vi "Celestial GOTO GUI.vi"() -> ()   [LabVIEW 2017]
uses:
  CaseEnum.ctl
  EventCase.ctl
  <vilib>/Instr/_visa.llb/VISA Configure Serial Port (Instr).vi
panel:
  out "DEC Angular Degrees":dbl[](array[numeric]) format="%#_4g"
  out "RA Angular Degrees":dbl[](array[numeric]) format="%#_4g"
  out "Source Coordinates RA/DE":T1
  in  "Source Target":u32(ring) items=["Mirach", "Mirphak", "Deneb", "Vega", "Sadr", "NGC6960", "M31", "M27", "M33", "M45", ""]
  in  "DEC-":bool
  in  "DEC+":bool
  in  "RA-":bool
  in  "RA+":bool
  in  "GOTO Destination":bool
  in  "VISA resource name":refnum<visa-resource-name>
  out "Serial Response":string
  out "Error Out":errorcluster
  out "Coordinate Difference (degrees)":cluster{"RA Degrees":dbl, "DE Degrees":dbl} {"DE Degrees" format="%#_3g"; "RA Degrees" format="%#_3g"}
  out "Destination Coordinates RA/DE":T1
  in  "Destination Target":u32(ring) items=["Mirach", "Mirphak", "Deneb", "Vega", "Sadr", "NGC6960", "M31", "M27", "M33", "M45", ""]
  in  "Stop Button":bool
  in  "Cluster":T2 {"Degrees to Move" format="%#_2g"}
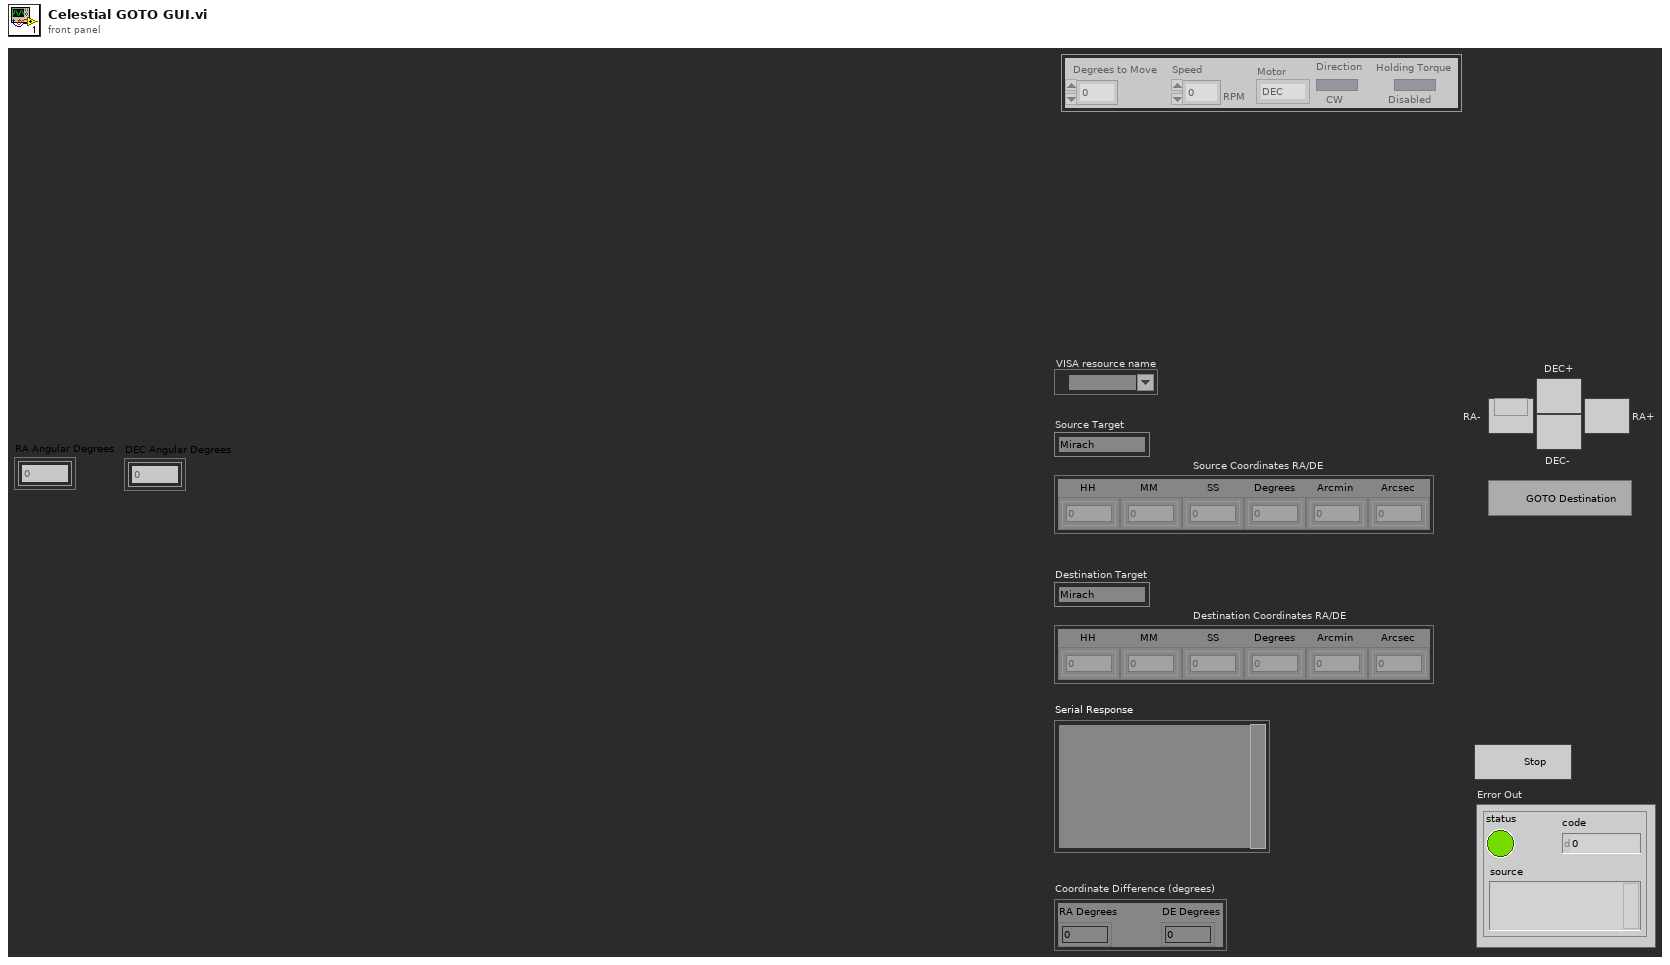
[diagram p1: front panel]
types:
  T1 = cluster{"HH":i32[], "MM":i32[], "SS":i32[], "Degrees":i32[], "Arcmin":i32[], "Arcsec":i32[]}
  T2 = cluster{"Degrees to Move":dbl, "Speed":i32, "Motor":enum16{"DEC", "RA"}, "Direction":bool, "Holding Torque":bool}
  T3 = typedef "CaseEnum.ctl" = enum16{"Default", "Parse Database", "Compute Coordinate Difference", "Move RA Motor", "Wait", "Move DEC Motor", "RA-", "RA+", "DEC-", "DEC+"}
  T4 = typedef "EventCase.ctl" = enum16{"Event", "Serial Write", "Wait", "Serial Read", "Stop"}
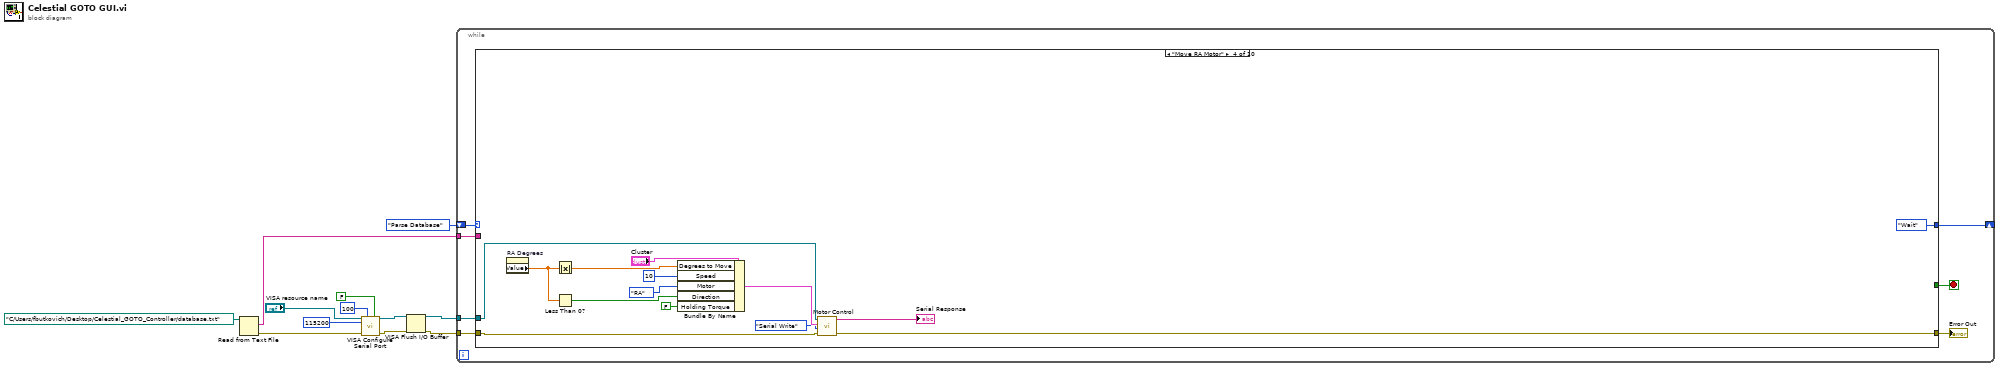
[diagram p0: block diagram]
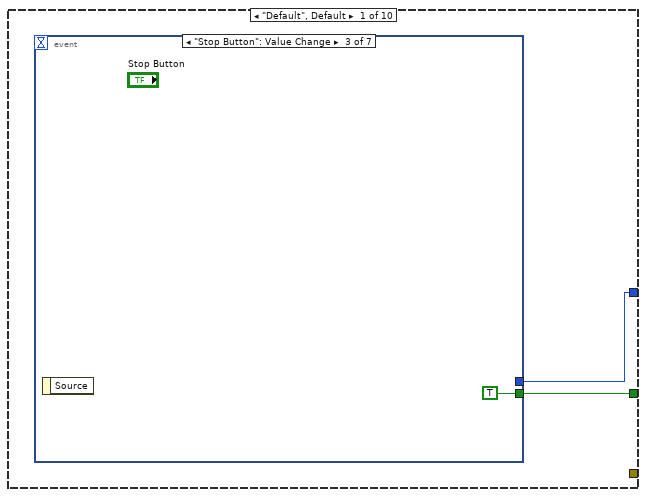
[diagram p2: hidden frame]
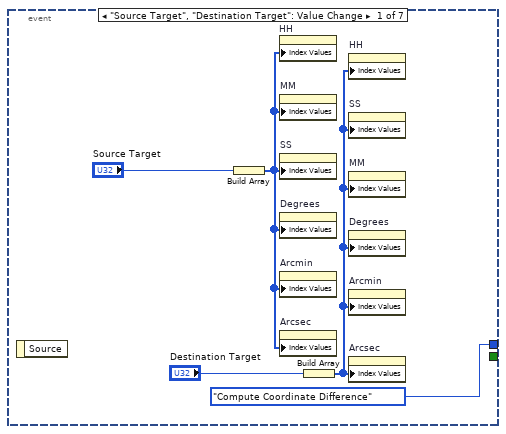
[diagram p3: hidden frame]
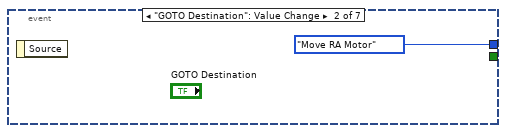
[diagram p4: hidden frame]
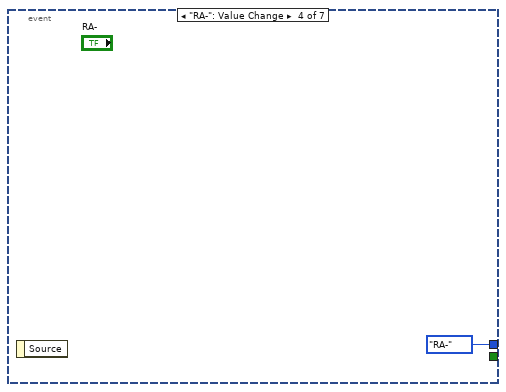
[diagram p5: hidden frame]
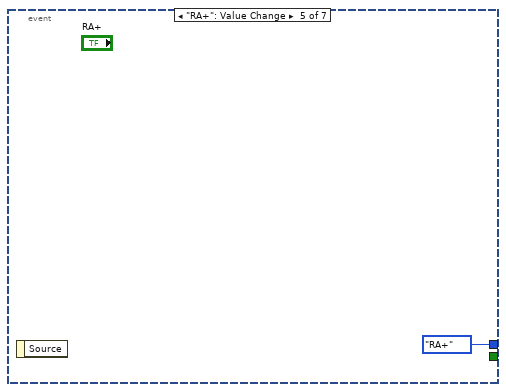
[diagram p6: hidden frame]
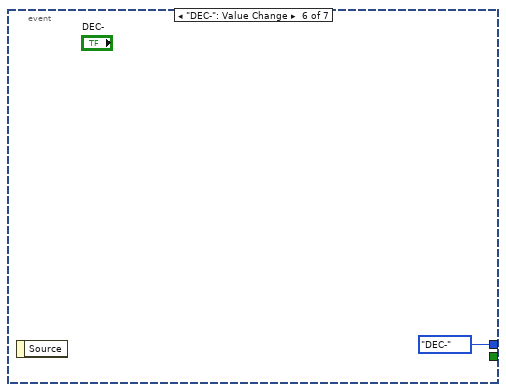
[diagram p7: hidden frame]
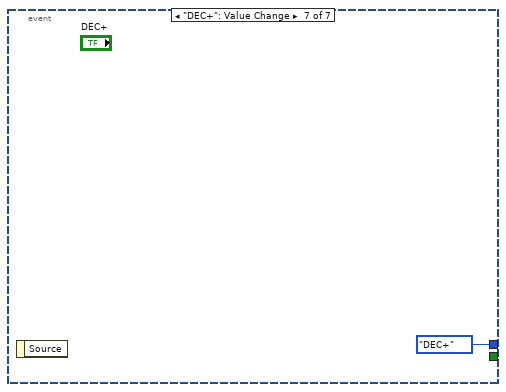
[diagram p8: hidden frame]
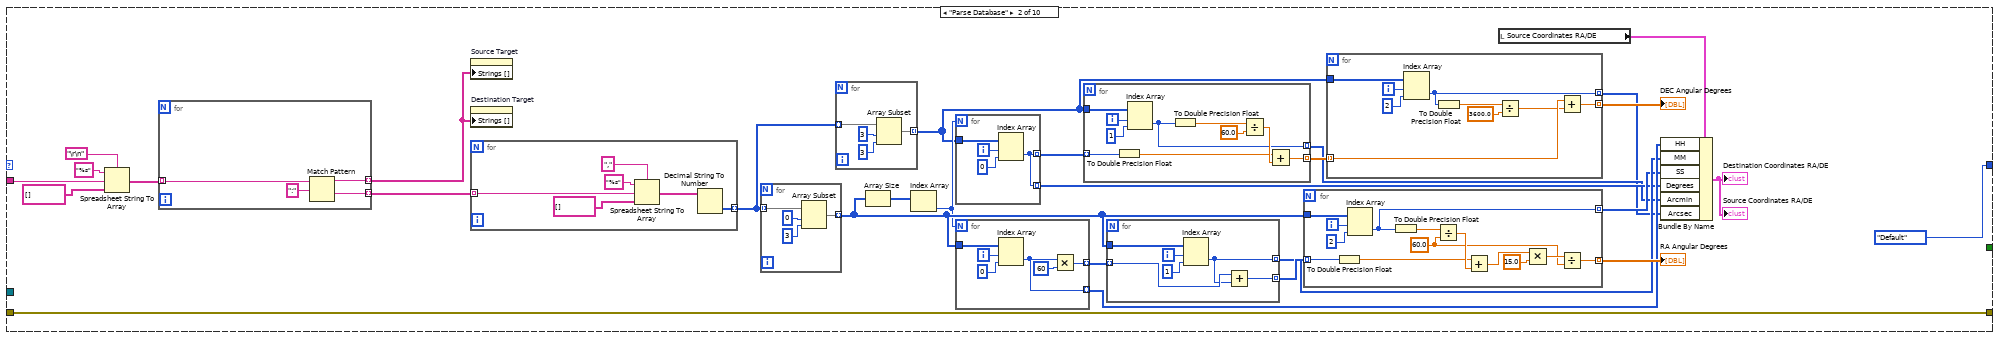
[diagram p9: hidden frame]
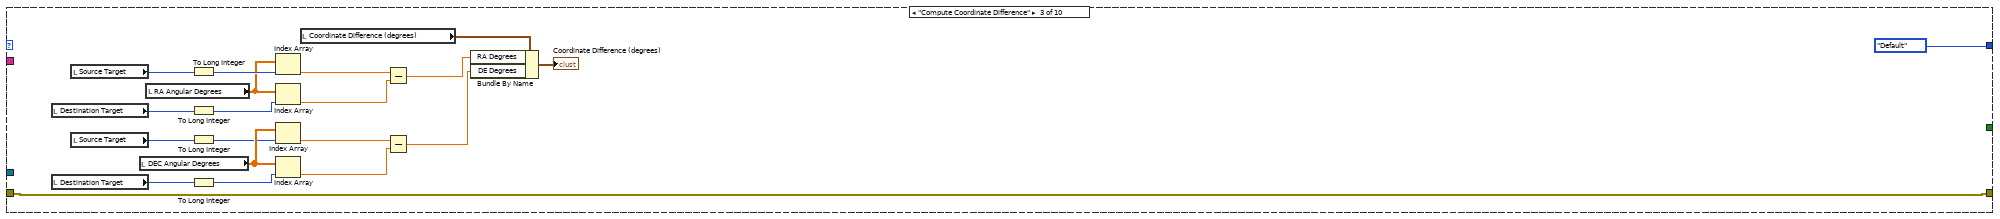
[diagram p10: hidden frame]
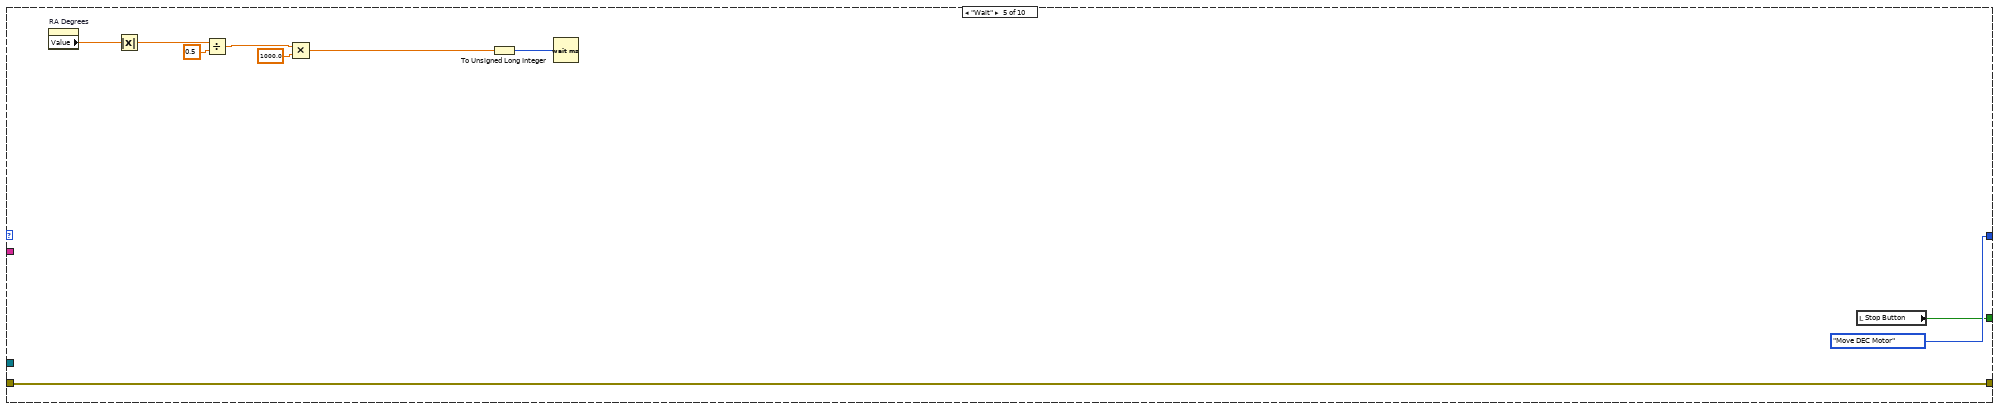
[diagram p11: hidden frame]
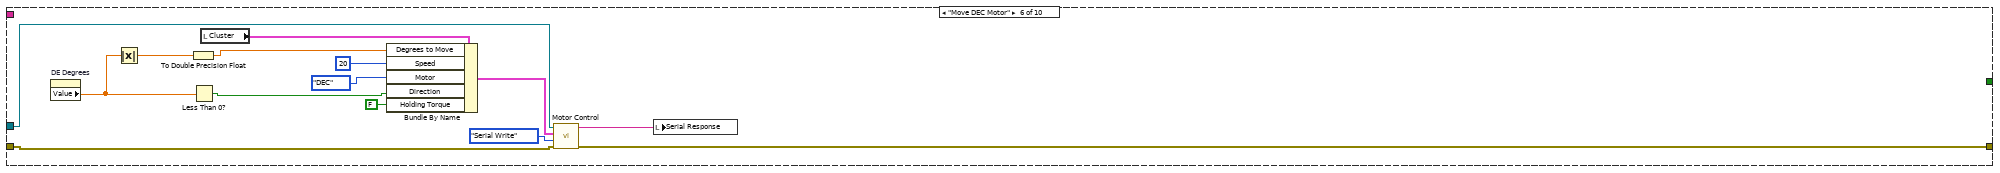
[diagram p12: hidden frame]
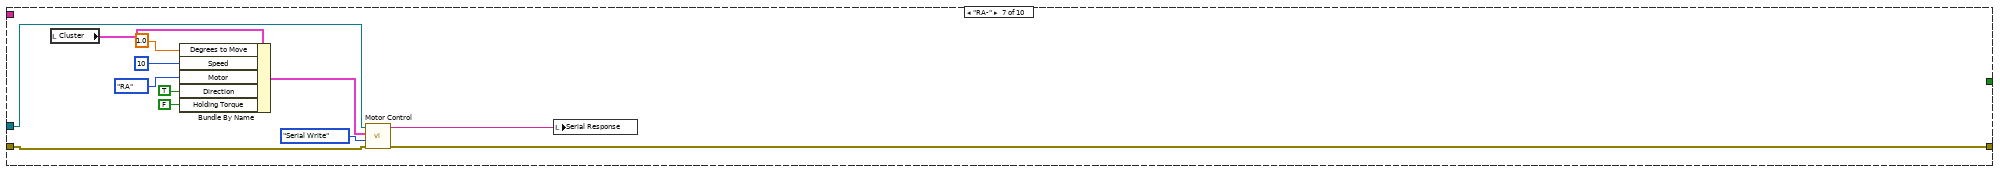
[diagram p13: hidden frame]
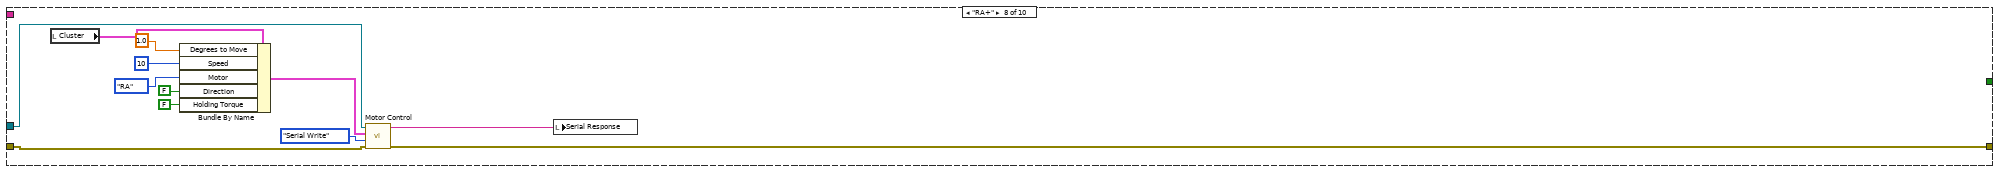
[diagram p14: hidden frame]
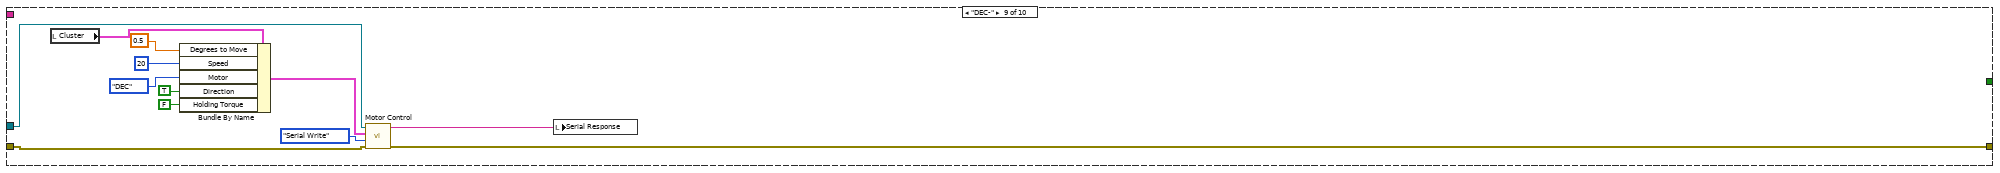
[diagram p15: hidden frame]
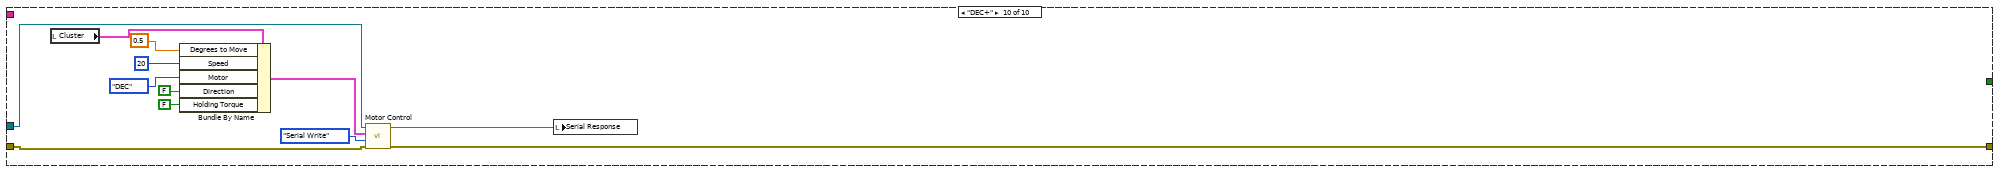
[diagram p16: hidden frame]
diagram:
  n1 = Read from Text File(file (use dialog)=path "C:/Users/fbutkovich/Desktop/Celestial_GOTO_Controller/database.txt" ("file path (use dialog)")) -> (text=w10:string, error out=w5:errorcluster)  [unwired: 3 in, 2 out]
  n2 = call-poly "VISA Configure Serial Port"("VISA resource name"="VISA resource name", "timeout (10sec)"=u32 100, "Enable Termination\nChar (T)"=FALSE, "baud rate (9600)"=u32 115200, "error in (no error)"=w5) -> ("VISA resource name out"=w6:refnum<visa-resource-name>, "error out"=w2:errorcluster)  [unwired: 9 in]
  n3 = VISA Flush I/O Buffer(VISA resource name=w6, error in (no error)=w2) -> (VISA resource name out=w3:refnum<visa-resource-name>, error out=w1:errorcluster)  [unwired: 1 in]
  n4 = while {
    tunnel: w10 -> [w17]
    tunnel: w1 -> [w15]
    shift-right: [w18] -> _
    shift-left: CaseEnum."Parse Database" -> [w19]
    tunnel: w3 -> [w13]
    stop <- w16 stop-if-true
    n5 = case shown="\"Move RA Motor\"" w19 {
      tunnel: [w21 CaseEnum."Default" CaseEnum."Default" CaseEnum."Wait" CaseEnum."Move DEC Motor" _ _ _ _ _] -> w18
      tunnel: w17 -> [_ w54 _ _ _ _ _ _ _ _]
      tunnel: [w20 _ _ _ w162 _ _ _ _ _] -> w16
      tunnel: [_ w59 w127 w159 w161 w184 w190 w197 w210 w224] -> w14
      tunnel: w15 -> [_ w59 w127 w148 w161 w173 w191 w201 w211 w225]
      tunnel: w13 -> [_ _ _ w150 _ w175 w192 w202 w212 w226]
      frame "Default", Default {
        n6 = event shown="[2] \"Stop Button\": Value Change" {
          selector: _ -> [_ _ _ _ _ _ _]
          dyn-events: _ -> [_ _ _ _ _ _ _]
          timeout: _ -> [_ _ _ _ _ _ _]
          tunnel: [CaseEnum."Compute Coordinate Difference" CaseEnum."Move RA Motor" _ CaseEnum."RA-" CaseEnum."RA+" CaseEnum."DEC-" CaseEnum."DEC+"] -> w21
          tunnel: [_ _ TRUE _ _ _ _] -> w20
          event "Source Target", "Destination Target": Value Change {
            n7 = event-data() -> ()  [unwired: 1 in, 1 out]
            n8 = Build Array("Source Target") -> (w22:u32[])
            n9 = property on="HH" class="Arr (strict)"("Index Values"=w22) -> ()  [unwired: 2 in, 2 out]
            n10 = property on="MM" class="Arr (strict)"("Index Values"=w22) -> ()  [unwired: 2 in, 2 out]
            n11 = property on="SS" class="Arr (strict)"("Index Values"=w22) -> ()  [unwired: 2 in, 2 out]
            n12 = property on="Degrees" class="Arr (strict)"("Index Values"=w22) -> ()  [unwired: 2 in, 2 out]
            n13 = property on="Arcmin" class="Arr (strict)"("Index Values"=w22) -> ()  [unwired: 2 in, 2 out]
            n14 = property on="Arcsec" class="Arr (strict)"("Index Values"=w22) -> ()  [unwired: 2 in, 2 out]
            n15 = Build Array("Destination Target") -> (w23:u32[])
            n16 = property on="HH" class="Arr (strict)"("Index Values"=w23) -> ()  [unwired: 2 in, 2 out]
            n17 = property on="SS" class="Arr (strict)"("Index Values"=w23) -> ()  [unwired: 2 in, 2 out]
            n18 = property on="MM" class="Arr (strict)"("Index Values"=w23) -> ()  [unwired: 2 in, 2 out]
            n19 = property on="Degrees" class="Arr (strict)"("Index Values"=w23) -> ()  [unwired: 2 in, 2 out]
            n20 = property on="Arcmin" class="Arr (strict)"("Index Values"=w23) -> ()  [unwired: 2 in, 2 out]
            n21 = property on="Arcsec" class="Arr (strict)"("Index Values"=w23) -> ()  [unwired: 2 in, 2 out]
          }
          event "GOTO Destination": Value Change {
            n22 = event-data() -> ()  [unwired: 1 in, 1 out]
          }
          event "Stop Button": Value Change {
            n23 = event-data() -> ()  [unwired: 1 in, 1 out]
          }
          event "RA-": Value Change {
            n24 = event-data() -> ()  [unwired: 1 in, 1 out]
          }
          event "RA+": Value Change {
            n25 = event-data() -> ()  [unwired: 1 in, 1 out]
          }
          event "DEC-": Value Change {
            n26 = event-data() -> ()  [unwired: 1 in, 1 out]
          }
          event "DEC+": Value Change {
            n27 = event-data() -> ()  [unwired: 1 in, 1 out]
          }
        }
      }
      frame "Parse Database" {
        n28 = Spreadsheet String To Array(delimiter (Tab)="\r\n", format string="%s", spreadsheet string=w54, array type (2D Dbl)=string[] []) -> (array=w55:string[])
        n29 = for {
          tunnel: w55 -> [w126] mode=indexing
          tunnel: [w124] -> w41 mode=indexing
          tunnel: [w123] -> w53 mode=indexing
          n30 = Match Pattern(string=w126, regular expression=":") -> (before substring=w123:string, after substring=w124:string)  [unwired: 1 in, 2 out]
        }
        n31 = property on="Source Target" class="Ring (strict)"("Strings []"=w53) -> ()  [unwired: 2 in, 2 out]
        n32 = property on="Destination Target" class="Ring (strict)"("Strings []"=w53) -> ()  [unwired: 2 in, 2 out]
        n33 = for {
          tunnel: [w118] -> w52 mode=indexing
          tunnel: w41 -> [w117] mode=indexing
          n34 = Spreadsheet String To Array(delimiter (Tab)=",", format string="%s", spreadsheet string=w117, array type (2D Dbl)=string[] []) -> (array=w119:string[])
          n35 = Decimal String To Number(string=w119) -> (number=w118:i32[])  [unwired: 2 in, 1 out]
        }
        n36 = for {
          tunnel: w52 -> [w116] mode=indexing
          tunnel: [w115] -> w49 mode=indexing
          n37 = Array Subset(array=w116, index=0, length=3) -> (w115:i32[])
        }
        n38 = for {
          tunnel: w52 -> [w112] mode=indexing
          tunnel: [w111] -> w44 mode=indexing
          n39 = Array Subset(array=w112, index=3, length=3) -> (w111:i32[])
        }
        n40 = Array Size(array=w49) -> (size(s)=w51:i32[])
        n41 = Index Array(array=w51) -> (element=w45:i32)  [unwired: 1 in]
        n42 = for {
          N: w45 -> [_]
          tunnel: w44 -> [w83]
          tunnel: [w80] -> w46 mode=indexing
          tunnel: [w80] -> w36 mode=indexing
          i -> [w82]
          n43 = Index Array(array=w83, index (row)=w82, index (col)=0 ("disabled index (col)")) -> (element=w80:i32)
        }
        n44 = for {
          N: w45 -> [_]
          tunnel: w49 -> [w108]
          tunnel: [w104] -> w50 mode=indexing
          tunnel: [w103] -> w39 mode=indexing
          i -> [w107]
          n45 = Index Array(array=w108, index (row)=w107, index (col)=0 ("disabled index (col)")) -> (element=w103:i32)
          n46 = Multiply(x=w103, y=60) -> (x*y=w104:i32)
        }
        n47 = for {
          tunnel: w44 -> [w78]
          tunnel: w46 -> [w77] mode=indexing
          tunnel: [w76] -> w43 mode=indexing
          tunnel: [w70] -> w35 mode=indexing
          i -> [w75]
          n48 = To Double Precision Float(number=w77) -> (double precision float=w71:dbl)
          n49 = Index Array(array=w78, index (row)=w75, index (col)=1) -> (element=w70:i32)
          n50 = To Double Precision Float(number=w70) -> (double precision float=w73:dbl)
          n51 = Divide(x=w73, y=60.0) -> (x/y=w72:dbl)
          n52 = Add(x=w71, y=w72) -> (x+y=w76:dbl)
        }
        n53 = for {
          tunnel: w49 -> [w101]
          tunnel: w50 -> [w100] mode=indexing
          tunnel: [w99] -> w48 mode=indexing
          tunnel: [w97] -> w38 mode=indexing
          i -> [w98]
          n54 = Index Array(array=w101, index (row)=w98, index (col)=1) -> (element=w97:i32)
          n55 = Add(x=w100, y=w97) -> (x+y=w99:i32)
        }
        n56 = for {
          tunnel: w49 -> [w95]
          tunnel: w48 -> [w94] mode=indexing
          tunnel: [w85] -> w47 mode=indexing
          tunnel: [w84] -> w37 mode=indexing
          i -> [w93]
          w86 = 60.0 ("y")
          n57 = To Double Precision Float(number=w94) -> (double precision float=w90:dbl)
          n58 = Index Array(array=w95, index (row)=w93, index (col)=2) -> (element=w84:i32)
          n59 = To Double Precision Float(number=w84) -> (double precision float=w92:dbl)
          n60 = Divide(x=w92, y=w86) -> (x/y=w91:dbl)
          n61 = Add(x=w90, y=w91) -> (x+y=w89:dbl)
          n62 = Multiply(x=w89, y=15.0) -> (x*y=w87:dbl)
          n63 = Divide(x=w87, y=w86) -> (x/y=w85:dbl)
        }
        "RA Angular Degrees" <- w47
        n64 = for {
          tunnel: w44 -> [w68]
          tunnel: w43 -> [w67] mode=indexing
          tunnel: [w66] -> w42 mode=indexing
          tunnel: [w61] -> w33 mode=indexing
          i -> [w65]
          n65 = Index Array(array=w68, index (row)=w65, index (col)=2) -> (element=w61:i32)
          n66 = To Double Precision Float(number=w61) -> (double precision float=w63:dbl)
          n67 = Divide(x=w63, y=3600.0) -> (x/y=w62:dbl)
          n68 = Add(x=w67, y=w62) -> (x+y=w66:dbl)
        }
        "DEC Angular Degrees" <- w42
        n69 = local read "Source Coordinates RA/DE"() -> (w40:T1)
        n70 = Bundle By Name(cluster=w40, "HH"=w39, "MM"=w38, "SS"=w37, "Degrees"=w36, "Arcmin"=w35, "Arcsec"=w33) -> (→"Destination Coordinates RA/DE" →"Source Coordinates RA/DE":T1)
      }
      frame "Compute Coordinate Difference" {
        n71 = local read "Destination Target"() -> (w138:u32)
        n72 = local read "Destination Target"() -> (w141:u32)
        n73 = local read "Source Target"() -> (w143:u32)
        n74 = local read "Source Target"() -> (w132:u32)
        n75 = local read "DEC Angular Degrees"() -> (w133:dbl[])
        n76 = local read "RA Angular Degrees"() -> (w136:dbl[])
        n77 = To Long Integer(number=w143) -> (32bit integer=w139:i32)
        n78 = To Long Integer(number=w138) -> (32bit integer=w137:i32)
        n79 = To Long Integer(number=w132) -> (32bit integer=w131:i32)
        n80 = To Long Integer(number=w141) -> (32bit integer=w140:i32)
        n81 = Index Array(array=w136, index=w139) -> (element=w142:dbl)
        n82 = Index Array(array=w136, index=w137) -> (element=w135:dbl)
        n83 = Index Array(array=w133, index=w131) -> (element=w130:dbl)
        n84 = Index Array(array=w133, index=w140) -> (element=w129:dbl)
        n85 = local read "Coordinate Difference (degrees)"() -> (w145:cluster{"RA Degrees":dbl, "DE Degrees":dbl})
        n86 = Subtract(x=w142, y=w135) -> (x-y=w134:dbl)
        n87 = Subtract(x=w130, y=w129) -> (x-y=w128:dbl)
        n88 = Bundle By Name(cluster=w145, "RA Degrees"=w134, "DE Degrees"=w128) -> (→"Coordinate Difference (degrees)":cluster{"RA Degrees":dbl, "DE Degrees":dbl})
      }
      frame "Move RA Motor" {
        n89 = property on="RA Degrees" class="DigNum (strict)"() -> ("Value"=w157:dbl)  [unwired: 2 in, 2 out]
        n90 = Absolute Value(x=w157) -> (abs(x)=w158:dbl)
        n91 = Less Than 0?(x=w157) -> (x < 0?=w156:bool)
        n92 = Bundle By Name(cluster="Cluster", "Degrees to Move"=w158, "Speed"=10, "Motor"=enum16{"DEC", "RA"}."RA", "Direction"=w156, "Holding Torque"=FALSE) -> (w149:T2)
        n93 = call "Motor Control.vi"("Error In"=w148, "Case Event"=EventCase."Serial Write", "Cluster"=w149, "VISA resource name"=w150) -> ("Error Out"=w159:errorcluster, "Serial Response"=→"Serial Response":string)  [unwired: 6 in]
      }
      frame "Wait" {
        n94 = property on="RA Degrees" class="DigNum (strict)"() -> ("Value"=w170:dbl)  [unwired: 2 in, 2 out]
        n95 = Absolute Value(x=w170) -> (abs(x)=w169:dbl)
        n96 = Divide(x=w169, y=0.5) -> (x/y=w167:dbl)
        n97 = Multiply(x=w167, y=1000.0) -> (x*y=w166:dbl)
        n98 = To Unsigned Long Integer(number=w166) -> (unsigned 32bit integer=w164:u32)
        n99 = Wait (ms)(milliseconds to wait=w164) -> ()  [unwired: 1 out]
        n100 = local read "Stop Button"() -> (w162:bool)
      }
      frame "Move DEC Motor" {
        n101 = property on="DE Degrees" class="DigNum (strict)"() -> ("Value"=w179:dbl)  [unwired: 2 in, 2 out]
        n102 = Absolute Value(x=w179) -> (abs(x)=w177:dbl)
        n103 = To Double Precision Float(number=w177) -> (double precision float=w178:dbl)
        n104 = Less Than 0?(x=w179) -> (x < 0?=w183:bool)
        n105 = local read "Cluster"() -> (w176:T2)
        n106 = Bundle By Name(cluster=w176, "Degrees to Move"=w178, "Speed"=20, "Motor"=enum16{"DEC", "RA"}."DEC", "Direction"=w183, "Holding Torque"=FALSE) -> (w174:T2)
        n107 = call "Motor Control.vi"("Error In"=w173, "Case Event"=EventCase."Serial Write", "Cluster"=w174, "VISA resource name"=w175) -> ("Error Out"=w184:errorcluster, "Serial Response"=w171:string)  [unwired: 6 in]
        n108 = local write "Serial Response"(w171) -> ()
      }
      frame "RA-" {
        n109 = local read "Cluster"() -> (w188:T2)
        n110 = Bundle By Name(cluster=w188, "Degrees to Move"=1.0, "Speed"=10, "Motor"=enum16{"DEC", "RA"}."RA", "Direction"=TRUE, "Holding Torque"=FALSE) -> (w187:T2)
        n111 = call "Motor Control.vi"("Error In"=w191, "Case Event"=EventCase."Serial Write", "Cluster"=w187, "VISA resource name"=w192) -> ("Error Out"=w190:errorcluster, "Serial Response"=w189:string)  [unwired: 6 in]
        n112 = local write "Serial Response"(w189) -> ()
      }
      frame "RA+" {
        n113 = local read "Cluster"() -> (w204:T2)
        n114 = Bundle By Name(cluster=w204, "Degrees to Move"=1.0, "Speed"=10, "Motor"=enum16{"DEC", "RA"}."RA", "Direction"=FALSE, "Holding Torque"=FALSE) -> (w203:T2)
        n115 = call "Motor Control.vi"("Error In"=w201, "Case Event"=EventCase."Serial Write", "Cluster"=w203, "VISA resource name"=w202) -> ("Error Out"=w197:errorcluster, "Serial Response"=w199:string)  [unwired: 6 in]
        n116 = local write "Serial Response"(w199) -> ()
      }
      frame "DEC-" {
        n117 = local read "Cluster"() -> (w214:T2)
        n118 = Bundle By Name(cluster=w214, "Degrees to Move"=0.5, "Speed"=20, "Motor"=enum16{"DEC", "RA"}."DEC", "Direction"=TRUE, "Holding Torque"=FALSE) -> (w213:T2)
        n119 = call "Motor Control.vi"("Error In"=w211, "Case Event"=EventCase."Serial Write", "Cluster"=w213, "VISA resource name"=w212) -> ("Error Out"=w210:errorcluster, "Serial Response"=w209:string)  [unwired: 6 in]
        n120 = local write "Serial Response"(w209) -> ()
      }
      frame "DEC+" {
        n121 = local read "Cluster"() -> (w222:T2)
        n122 = Bundle By Name(cluster=w222, "Degrees to Move"=0.5, "Speed"=20, "Motor"=enum16{"DEC", "RA"}."DEC", "Direction"=FALSE, "Holding Torque"=FALSE) -> (w223:T2)
        n123 = call "Motor Control.vi"("Error In"=w225, "Case Event"=EventCase."Serial Write", "Cluster"=w223, "VISA resource name"=w226) -> ("Error Out"=w224:errorcluster, "Serial Response"=w221:string)  [unwired: 6 in]
        n124 = local write "Serial Response"(w221) -> ()
      }
    }
    "Error Out" <- w14
  }
